vi "Port D_A Scan Step.vi"(7 "Read Value? (F)":bool, 8 "error in (no error)":errorcluster, 9 "Port Scan Step (0.000 V)":dbl format="%.3g", 10 "Port (1)":T1=enum."1", 11 "VISA resource name":refnum<visa-resource-name>) -> (0 "error out":errorcluster, 1 "Port Scan Step":dbl format="%.3g", 3 "VISA resource name out":refnum<visa-resource-name>)   [LabVIEW 2013, in "SRS SR400.lvlib"]
doc: "<B>PY i { ,v }</B>\n\nThe PY command sets and reads the PORT1 and PORT2 scan steps. i=1 or 2 to select PORT1 or PORT 2 and is required. If v is included, the scan step is set to v Volts where -0.500 <= v <= 0.500. The resolution is 0.005 V (5 mV). If v is absent, the scan step is returned. The scan step may be set and read even if the selected port is in the FIXED mode. Changing the scan step during a scan will affect the level for the next count period and all those that follow."
uses:
  <instrlib>/SRS SR400/SRS SR400.lvlib
  <instrlib>/SRS SR400/Public/Typedefs/Port.ctl
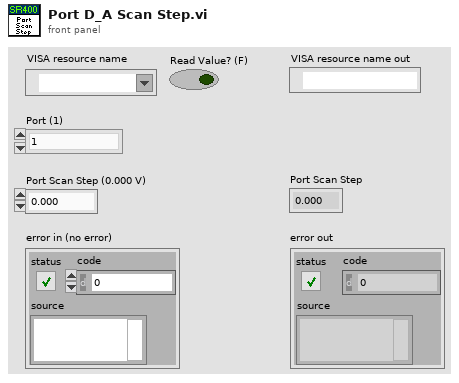
[diagram p1: front panel]
types:
  T1 = typedef "SRS SR400.lvlib/Port.ctl" = enum16{"(not used)", "1", "2"}
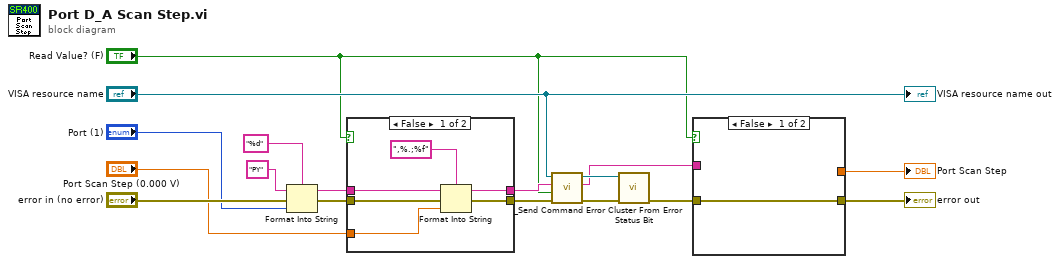
[diagram p0: block diagram]
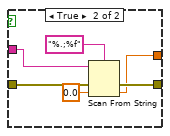
[diagram p2: hidden frame]
diagram:
  n1 = Format Into String(format string="%d", initial string="PY" ("command"), error in="error in (no error)", "Port (1)") -> (resulting string=w15:string, error out=w16:errorcluster)
  n2 = case shown="False" "Read Value? (F)" {
    tunnel: w16 -> [w23 w24]
    tunnel: w15 -> [w18 w25]
    tunnel: "Port Scan Step (0.000 V)" -> [w22 _]
    tunnel: [w20 w25] -> w11
    tunnel: [w19 w24] -> w10
    frame False {
      n3 = Format Into String(format string=",%.;%f", initial string=w18, error in=w23, w22) -> (resulting string=w20:string, error out=w19:errorcluster)
    }
    frame True {
    }
  }
  n4 = call <instrlib>:"_Send Command.vi"("error in (no error)"=w10, "Read Value? (F)"="Read Value? (F)", "Command"=w11, "VISA resource name"="VISA resource name") -> ("error out"=w6:errorcluster, "Response"=w3:string, "VISA resource name out"=w7:refnum<visa-resource-name>)  [unwired: 5 out]
  n5 = call <instrlib>:"Error Cluster From Error Status Bit.vi"("error in (no error)"=w6, "VISA resource name"=w7) -> ("error out"=w5:errorcluster)  [unwired: 8 in, 1 out]
  n6 = case shown="False" "Read Value? (F)" {
    tunnel: w5 -> [w26 w32]
    tunnel: [w26 w31] -> w4
    tunnel: w3 -> [_ w29]
    tunnel: [_ w27] -> w1
    frame False {
    }
    frame True {
      n7 = Scan From String(format string="%.;%f", input string=w29, error in=w32, default 1=0.0 ("default value 1")) -> (error out=w31:errorcluster, output 1=w27:dbl)  [unwired: 1 in, 2 out]
    }
  }
  "error out" <- w4
  "Port Scan Step" <- w1
  "VISA resource name out" <- "VISA resource name"
